vi "GLOBAL Z.vi"(10 "wZ":dbl, 11 "sZ":dbl) -> (2 "TZ":dbl)   [LabVIEW 2018]
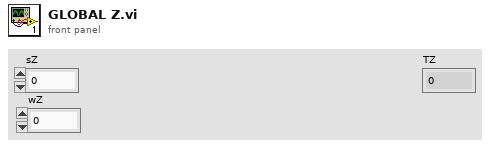
[diagram p1: front panel]
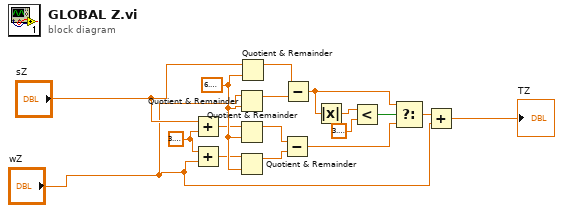
[diagram p0: block diagram]
diagram:
  w7 = 6.283185307179586
  w4 = 3.141592653589793
  n1 = Add(x="sZ", y=w4) -> (x+y=w5:dbl)
  n2 = Add(x=w4, y="wZ") -> (x+y=w6:dbl)
  n3 = Quotient & Remainder(x="wZ", y=w7) -> (x-y*floor(x/y)=w9:dbl)  [unwired: 1 out]
  n4 = Quotient & Remainder(x=w5, y=w7) -> (x-y*floor(x/y)=w10:dbl)  [unwired: 1 out]
  n5 = Quotient & Remainder(x=w6, y=w7) -> (x-y*floor(x/y)=w11:dbl)  [unwired: 1 out]
  n6 = Quotient & Remainder(x="sZ", y=w7) -> (x-y*floor(x/y)=w8:dbl)  [unwired: 1 out]
  n7 = Subtract(x=w10, y=w11) -> (x-y=w16:dbl)
  n8 = Subtract(x=w8, y=w9) -> (x-y=w15:dbl)
  n9 = Absolute Value(x=w15) -> (abs(x)=w12:dbl)
  n10 = Less?(x=w12, y=3.141592653589793) -> (x < y?=w14:bool)
  n11 = Select(t=w15, s=w14, f=w16) -> (s? t:f=w17:dbl)
  n12 = Add(x=w17, y="wZ") -> (x+y=→"TZ":dbl)
